vi "TCP_IP_N6705B_Press_Run_stop_button.vi"(8 "error in (no error)":errorcluster, 11 "instrument address":string) -> (0 "error out":errorcluster)   [LabVIEW 2015]
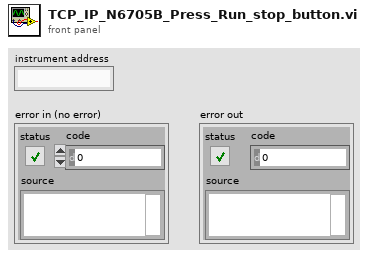
[diagram p1: front panel]
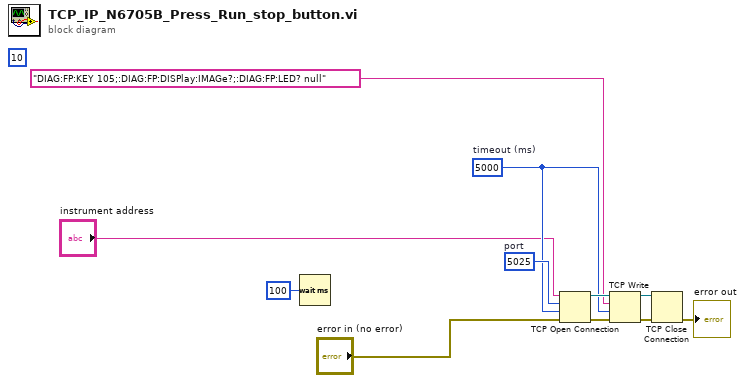
[diagram p0: block diagram]
diagram:
  w8 = u16 5025  # port
  w5 = 5000  # timeout (ms)
  (unwired) 10
  n1 = Wait (ms)(milliseconds to wait=u32 100) -> ()  [unwired: 1 out]
  n2 = TCP Open Connection(address="instrument address", remote port or service name=w8, timeout ms (60000)=w5, error in (no error)="error in (no error)") -> (connection ID=w9:refnum<k5>, error out=w10:errorcluster)  [unwired: 1 in]
  n3 = TCP Write(connection ID=w9, data in="DIAG:FP:KEY 105;:DIAG:FP:DISPlay:IMAGe?;:DIAG:FP:LED? null" ("Back  2"), error in (no error)=w10, 9:w5) -> (connection ID out=w6:refnum<k5>, error out=w7:errorcluster)  [unwired: 1 out]
  n4 = TCP Close Connection(connection ID=w6, error in (no error)=w7) -> (error out=→"error out":errorcluster)  [unwired: 1 in, 1 out]
